vi "LOCATORMOD.vi"() -> ()   [LabVIEW 2009]
uses:
  <vilib>/Utility/file.llb/Read From Spreadsheet File (string).vi
  <vilib>/Utility/file.llb/Write To Spreadsheet File (string).vi
panel:
  out "subarray":string[](array[string])
  out "Found?":bool
  out "Array":string[][](array[string])
  in  "Pillar":string
  in  "Store":bool
  in  "Search":bool
  in  "Car Number":string
  in  "stop":bool
  out "index":i32
  in  "file path (use dialog)":path=path "C:/Users/Bill/Desktop/TESTCAR1.txt"
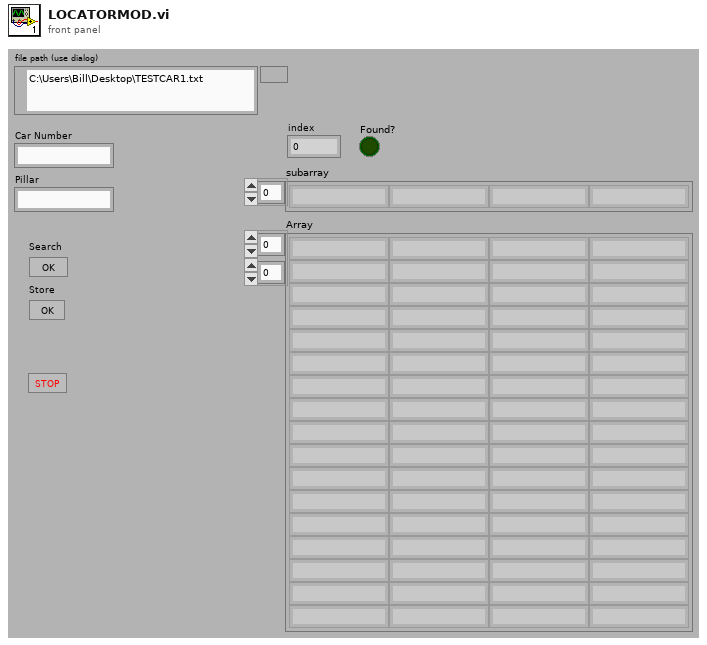
[diagram p1: front panel]
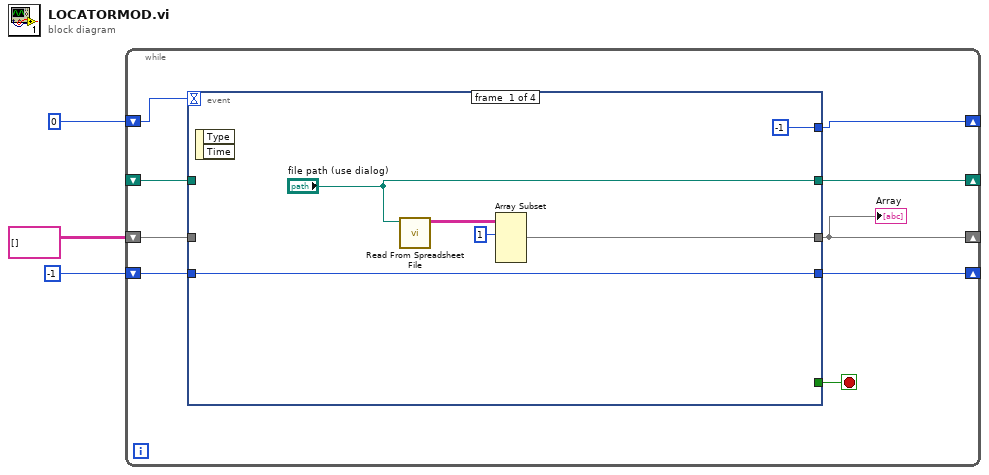
[diagram p0: block diagram]
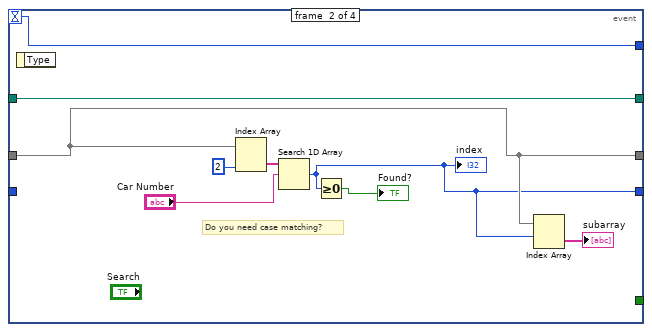
[diagram p2: hidden frame]
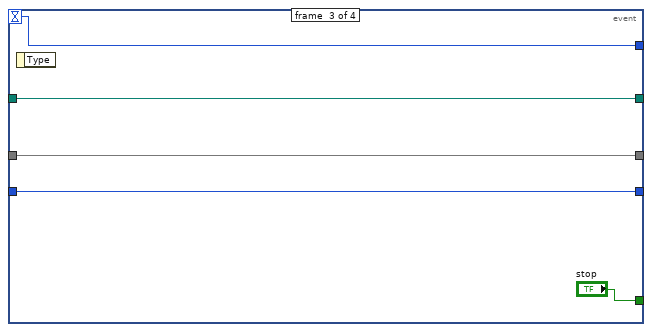
[diagram p3: hidden frame]
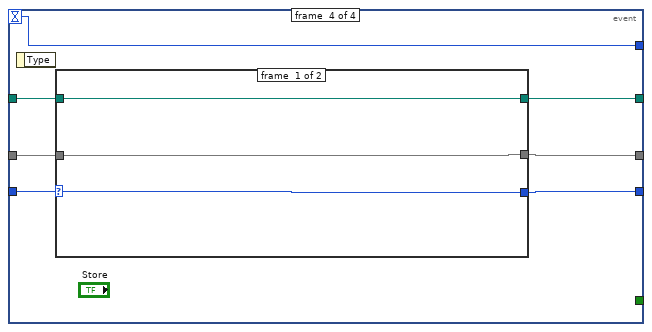
[diagram p4: hidden frame]
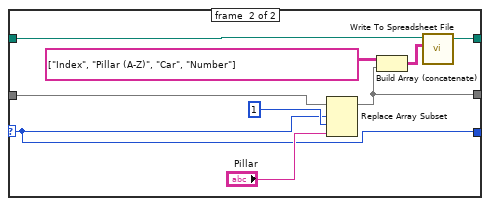
[diagram p5: hidden frame]
diagram:
  n1 = while {
    shift-right: [w11] -> _
    shift-left: 0 -> [w12]
    shift-right: [w10] -> _
    shift-left: _ -> [w7]
    shift-right: [w9] -> _
    shift-left: string[][] [] -> [w8]
    shift-right: [w6] -> _
    shift-left: -1 ("index of element") -> [w5]
    stop <- w4 stop-if-true
    n2 = event shown="[3] \"Store\": Value Change" {
      selector: _ -> [_ _ _ _]
      dyn-events: _ -> [_ _ _ _]
      timeout: w12 -> [_ w23 w32 w33]
      tunnel: [-1 w23 w32 w33] -> w11
      tunnel: ["file path (use dialog)" w24 w31 w34] -> w10
      tunnel: [w14 w21 w30 w38] -> w9
      tunnel: w8 -> [_ w21 w30 w39]
      tunnel: w7 -> [_ w24 w31 w35]
      tunnel: [w13 w20 w29 w36] -> w6
      tunnel: w5 -> [w13 _ w29 w37]
      tunnel: [_ _ "stop" _] -> w4
      event #0 {
        n3 = event-data() -> ()  [unwired: 1 in, 2 out]
        n4 = call-poly <vilib>:"Read From Spreadsheet File.vi"("file path (dialog if empty)"="file path (use dialog)") -> ("all rows"=w16:string[][])  [unwired: 6 in, 4 out]
        n5 = Array Subset(array=w16, index (row)=1 ("index")) -> (w14:string[][])  [unwired: 3 in]
      }
      event #1 {
        # "Do you need case matching?"
        n6 = event-data() -> ()  [unwired: 1 in, 1 out]
        n7 = Index Array(array=w21, index (col)=2 ("disabled index (col)")) -> (element=w26:string[])  [unwired: 1 in]
        n8 = Search 1D Array(1D array=w26, element="Car Number") -> (index of element=w20:i32)  [unwired: 1 in]
        "index" <- w20
        n9 = Greater Or Equal To 0?(x=w20) -> (x >= 0?=→"Found?":bool)
        n10 = Index Array(array=w21, index (row)=w20) -> (element=→"subarray":string[])  [unwired: 1 in]
      }
      event #2 {
        n11 = event-data() -> ()  [unwired: 1 in, 1 out]
      }
      event #3 {
        n12 = event-data() -> ()  [unwired: 1 in, 1 out]
        n13 = case shown="Default" w37 {
          selector: w37 -> [w41 w48]
          tunnel: w39 -> [w42 w51]
          tunnel: [w42 w43] -> w38
          tunnel: [w41 w48] -> w36
          tunnel: w35 -> [w40 w47]
          tunnel: [w40 w46] -> w34
          frame #0 {
          }
          frame #1 {
            n14 = Replace Array Subset(array=w51, new element="Pillar", index (row)=w48, index (col)=1 ("disabled index (col)")) -> (w43:string[][])
            n15 = Build Array (concatenate)(string[][] [["Index", "Pillar (A-Z)", "Car", "Number"]] ("output array"), w43) -> (w44:string[][])
            n16 = call-poly <vilib>:"Write To Spreadsheet File.vi"("2D data"=w44, "file path (dialog if empty)"=w47) -> ("new file path (Not A Path if cancelled)"=w46:path)  [unwired: 6 in]
          }
        }
      }
    }
    "Array" <- w9
  }
